vi "Waveform Buffer Generation.vi"(5 "Amplitude":dbl=2.0 format="%0.2p", 6 "Cycles per Buffer":dbl=1.0 format="%.2f", 7 "Samples per Buffer":dbl=1000.0, 8 "error in":errorcluster caption="error in (no error)", 9 "Waveform Type":u16(ring) items=["Sine Wave", "Triangle Wave", "Square Wave", "Sawtooth Wave"], 10 "Desired Frequency":dbl=1000.0 format="%.2f", 11 "task/channels in":refnum<k21>) -> (0 "error out":errorcluster, 1 "Resulting Frequency":dbl format="%.2f", 2 "Waveform":waveform(dbl), 3 "task out":refnum<k21>, 4 "Resulting Sample Clock Rate":dbl format="%.2f")   [LabVIEW 2022 SP3]
doc: "This subVI is used to create a Sine, Square, Triangle or Sawtooth Waveform. The inputs to this VI are the Waveform Type, which determines if the output waveform is a Sine, Square, Triangle, or Sawtooth Waveform, the amplitude, Desired Frequency, Samples per Buffer, and Cycles per Buffer. \n\nThe Desired Frequency, Samples per Buffer, and Cycles per Buffer are used to calculate the sample clock rate. The DAQmx Timing property node sets the sample clock rate for the device specified in the task/channels in control. \n\nThe actual, coerced, sample clock rate is returned and used as an input to the Basic Function Generator.vi. The Basic Function Generator returns a waveform of data with timing information.\n\nThe formula below was used to determine the sample clock rate:\n\nDesired Frequency=[(Cycles/Buffer)X(Sample Clock Rate)]/Samples per Buffer\n\nNote: The Block Diagram rearranges the variables to solve for Sample Clock Rate"
uses:
  <vilib>/measure/NI_MABase.lvlib
  <resource>/objmgr/daqmx.rc
panel:
  out "Samples/cycle":dbl format="%0.2f"
  out "Desired Sample Clock Rate":dbl format="%.2f"
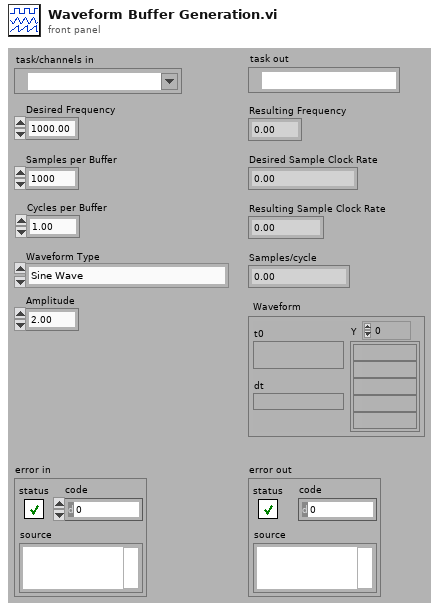
[diagram p1: front panel]
types:
  T1 = cluster{"SampleTakt.Rate":dbl, "Samples per Buffer":dbl}
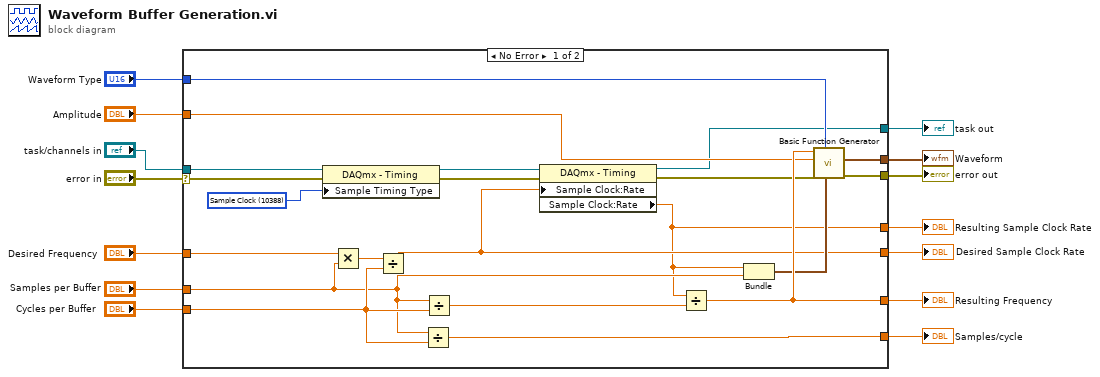
[diagram p0: block diagram]
diagram:
  n1 = case shown="No Error" "error in" {
    selector: "error in" -> [w15 w37]
    tunnel: [w35 _] -> w14
    tunnel: "Desired Frequency" -> [w34 _]
    tunnel: [w32 _] -> w12
    tunnel: [w30 _] -> w11
    tunnel: "Cycles per Buffer" -> [w29 _]
    tunnel: [w27 _] -> w9
    tunnel: "Waveform Type" -> [w26 _]
    tunnel: "Amplitude" -> [w25 _]
    tunnel: "Samples per Buffer" -> [w24 _]
    tunnel: [w23 w36] -> w5
    tunnel: [w22 _] -> w4
    tunnel: [w20 w37] -> w3
    tunnel: "task/channels in" -> [w16 w36]
    frame No Error {
      w17 = 10388 items=["Sample Clock"=10388, "Handshake"=10389, "Implicit"=10451, "On Demand"=10390, "Change Detection"=12504] ("SampTimingType")
      n2 = property class="DAQmx - Timing"(reference=w16, error in=w15, "Sample Timing Type"=w17) -> (reference out=w19:refnum<k21>, error out=w18:errorcluster)
      n3 = Multiply(x=w34, y=w24) -> (x*y=w31:dbl)
      n4 = Divide(x=w31, y=w29) -> (x/y=w27:dbl)
      n5 = Divide(x=w24, y=w29) -> (x/y=w30:dbl)
      n6 = Divide(x=w24, y=w29) -> (x/y=w28:dbl)
      n7 = property class="DAQmx - Timing"(reference=w19, error in=w18, "Sample Clock:Rate"=w27) -> (reference out=w23:refnum<k21>, error out=w21:errorcluster, "Sample Clock:Rate"=w22:dbl)
      n8 = Divide(x=w22, y=w28) -> (x/y=w35:dbl)
      n9 = Bundle("SampleTakt.Rate"=w22, "Samples per Buffer"=w24) -> (w33:T1)  [unwired: 1 in]
      n10 = call <vilib>:"Basic Function Generator.vi"("sampling info"=w33, "signal type"=w26, "error in (no error)"=w21, "amplitude"=w25, "frequency"=w35) -> ("error out"=w20:errorcluster, "signal out"=w32:waveform(dbl))  [unwired: 4 in, 1 out]
    }
    frame Error {
    }
  }
  "Resulting Sample Clock Rate" <- w4
  "Desired Sample Clock Rate" <- w9
  "Resulting Frequency" <- w14
  "Waveform" <- w12
  "Samples/cycle" <- w11
  "error out" <- w3
  "task out" <- w5
